vi "Load-Save Hardware Config.vi"(7 "Standalone ?":bool, 8 "error in":errorcluster, 9 "Hardware Configuration I/P":T1={"Dev. PC"=FALSE, "Swap XY on stage"=FALSE, "No of AOD"=0, "Computer MAC address"="", "Externalise Triggers"=FALSE, "Trigger HW config"={"Available Device List"=0, "Device Address"=""}, "DAQmx Chan"={"Pockels AO"="", "Hard shutter AO"="", "PMT AOs"="", "Galvo AOs"="", "Power meter AI"=""}, "XY stage available"=FALSE, "XY Stage"={"COM port"="", "Baudrate"=0, "Type"=""}, "Z stage available"=FALSE, "Z Stage config cluster"={"COM port"="COM7", "Baudrate"=0, "Type"=""}, "Encoder available"=FALSE, "Encoder"={"IP address"="224.0.1.103", "Port"=7000, "Wheel radius (cm)"=16.0, "Encoder Trigger"=""}, "VidRec available"=FALSE, "Cam VidRec"={"DO flag-Video record"="", "DO flag-Trial start"=""}, "Laser Power Control HW config"={"Laser Power Control"="", "Laser Power Modulation Control"=enum."NI"}, "Laser 1 available"=FALSE, "Laser 1 config cluster"={"COM port"="COM7", "Baud Rate"=0, "Type"=""}, "Prechirper 1 available"=FALSE, "Prechirper 1 config cluster"={"Type"="", "Baud Rate"=0, "COM port"="COM7"}, "Control system.FPGA available?"=FALSE, "Control Sys. HW config"={"Control system.FPGA Type"=enum."Virtex 5", "Control system.Network adapter name"="", "Control system.MAC address"="", "Control system.Ethernet Port"=0, "Control system.Ethernet Port Opened"=FALSE}, "DAQ FPGA HW Config"={"FGPA Ref"=refnum, "Target"="RIO0", "input card type"=enum."AC Card"}} {"Encoder"."Wheel radius (cm)" format="%#_13g"}, 11 "Function":T16=enum."Load from file") -> (0 "error out":errorcluster, 1 "Hardware Configuration O/P":T1={"Dev. PC"=FALSE, "Swap XY on stage"=FALSE, "No of AOD"=0, "Computer MAC address"="", "Externalise Triggers"=FALSE, "Trigger HW config"={"Available Device List"=0, "Device Address"=""}, "DAQmx Chan"={"Pockels AO"="", "Hard shutter AO"="", "PMT AOs"="", "Galvo AOs"="", "Power meter AI"=""}, "XY stage available"=FALSE, "XY Stage"={"COM port"="", "Baudrate"=0, "Type"=""}, "Z stage available"=FALSE, "Z Stage config cluster"={"COM port"="COM7", "Baudrate"=0, "Type"=""}, "Encoder available"=FALSE, "Encoder"={"IP address"="224.0.1.103", "Port"=7000, "Wheel radius (cm)"=16.0, "Encoder Trigger"=""}, "VidRec available"=FALSE, "Cam VidRec"={"DO flag-Video record"="", "DO flag-Trial start"=""}, "Laser Power Control HW config"={"Laser Power Control"="", "Laser Power Modulation Control"=enum."NI"}, "Laser 1 available"=FALSE, "Laser 1 config cluster"={"COM port"="COM7", "Baud Rate"=0, "Type"=""}, "Prechirper 1 available"=FALSE, "Prechirper 1 config cluster"={"Type"="", "Baud Rate"=0, "COM port"="COM7"}, "Control system.FPGA available?"=FALSE, "Control Sys. HW config"={"Control system.FPGA Type"=enum."Virtex 5", "Control system.Network adapter name"="", "Control system.MAC address"="", "Control system.Ethernet Port"=0, "Control system.Ethernet Port Opened"=FALSE}, "DAQ FPGA HW Config"={"FGPA Ref"=refnum, "Target"="RIO0", "input card type"=enum."AC Card"}} {"Encoder"."Wheel radius (cm)" format="%#_13g"})   [LabVIEW 2017]
uses:
  <vilib>/Utility/config.llb/NI_LVConfig.lvlib
  Typedefs/Which path.ctl
  Typedefs/XY Stage config cluster.ctl
  <vilib>/userdefined/High Color/nirio_resource_hc.ctl
  Typedefs/DAQmx physical channels cluster.ctl
  Typedefs/Save-Load enum.ctl
  Typedefs/FPGA input type AC-DC.ctl
  Typedefs/Encoder config cluster.ctl
  Typedefs/Cam VidRec HW config setup cluster.ctl
  Typedefs/Control Sys HW config cluster.ctl
  Typedefs/Z Stage config cluster.ctl
  Typedefs/Triggers HW config.ctl
  Typedefs/Laser 1 config cluster.ctl
  Typedefs/PreChirper 1 config cluster.ctl
  Typedefs/Laser Power Control HW config.ctl
  Typedefs/Hardware Configuration settings.ctl
  RIG-SPECIFIC FILES/FPGA Refs/FPGA Ref.ctl
  Typedefs/DAQ FPGA HW config cluster.ctl
panel:
  # "<--- The \"PMT AOs\" DAQmx string will always contain\n                       2 channels is this format: PXI1Slot4/ao2:3"
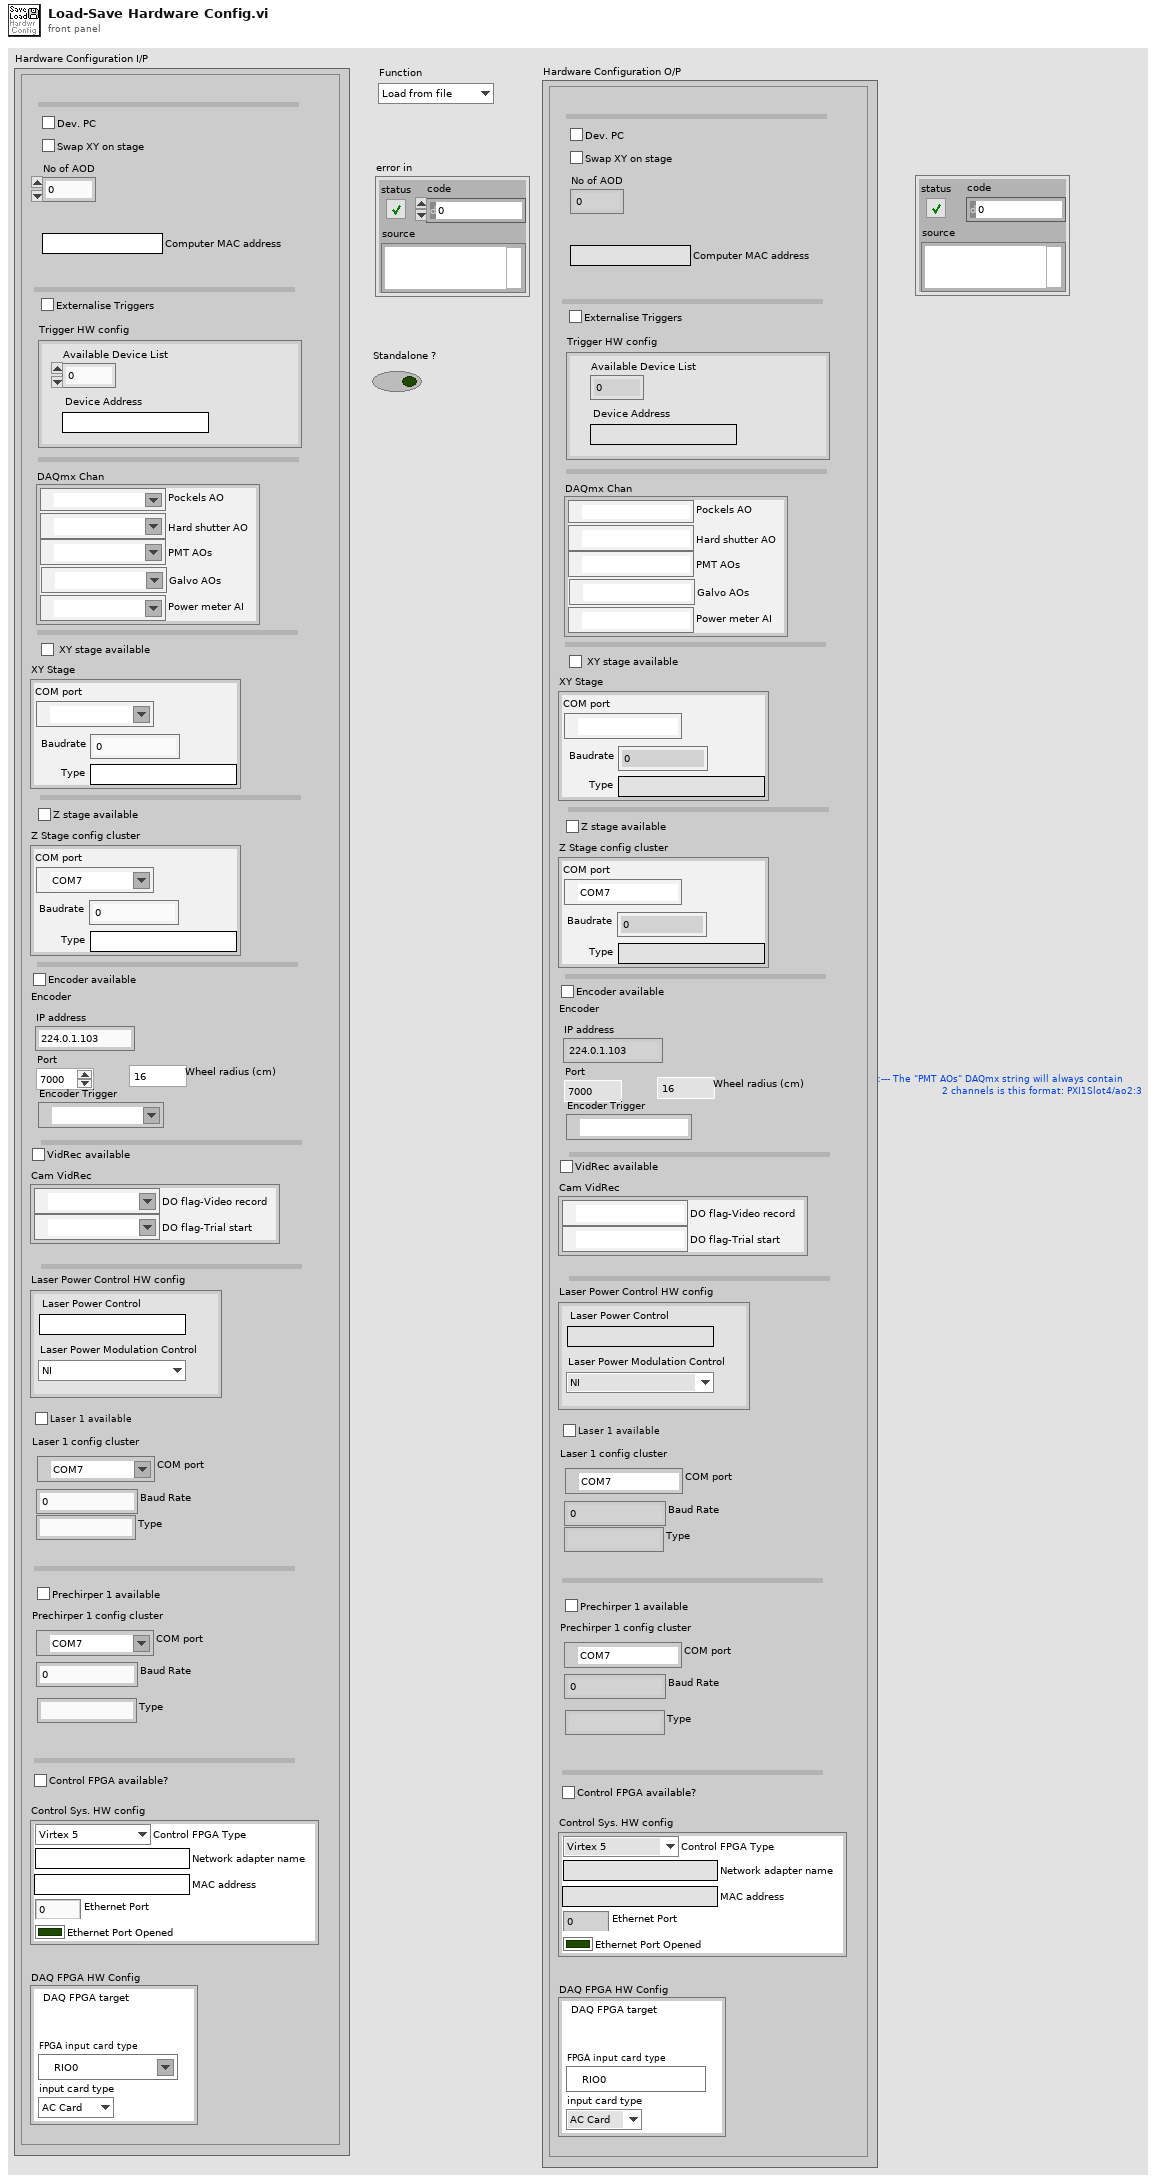
[diagram p1: front panel]
types:
  T1 = typedef "Hardware Configuration settings.ctl" = cluster{"Dev. PC":bool, "Swap XY on stage":bool, "No of AOD":u8, "Computer MAC address":string, "Externalise Triggers":bool, "Trigger HW config":T2, "DAQmx Chan":T3, "XY stage available":bool, "XY Stage":T4, "Z stage available":bool, "Z Stage config cluster":T5, "Encoder available":bool, "Encoder":T6, "VidRec available":bool, "Cam VidRec":T7, "Laser Power Control HW config":T8, "Laser 1 available":bool, "Laser 1 config cluster":T9, "Prechirper 1 available":bool, "Prechirper 1 config cluster":T10, "Control system.FPGA available?":bool, "Control Sys. HW config":T11, "DAQ FPGA HW Config":T12}
  T2 = typedef "Triggers HW config.ctl" = cluster{"Available Device List":i32, "Device Address":string}
  T3 = typedef "DAQmx physical channels cluster.ctl" = cluster{"Pockels AO":tag, "Hard shutter AO":tag, "PMT AOs":tag, "Galvo AOs":tag, "Power meter AI":tag}
  T4 = typedef "XY Stage config cluster.ctl" = cluster{"COM port":refnum<visa-resource-name>, "Baudrate":i32, "Type":string}
  T5 = typedef "Z Stage config cluster.ctl" = cluster{"COM port":refnum<visa-resource-name>, "Baudrate":i32, "Type":string}
  T6 = typedef "Encoder config cluster.ctl" = cluster{"IP address":string, "Port":u16, "Wheel radius (cm)":dbl, "Encoder Trigger":tag}
  T7 = typedef "Cam VidRec HW config setup cluster.ctl" = cluster{"DO flag-Video record":tag, "DO flag-Trial start":tag}
  T8 = typedef "Laser Power Control HW config.ctl" = cluster{"Laser Power Control":string, "Laser Power Modulation Control":enum16{"NI", "FPGA"}}
  T9 = typedef "Laser 1 config cluster.ctl" = cluster{"COM port":refnum<visa-resource-name>, "Baud Rate":i32, "Type":string}
  T10 = typedef "PreChirper 1 config cluster.ctl" = cluster{"Type":string, "Baud Rate":i32, "COM port":refnum<visa-resource-name>}
  T11 = typedef "Control Sys HW config cluster.ctl" = cluster{"Control system.FPGA Type":enum16{"Virtex 5", "Virtex 7"}, "Control system.Network adapter name":string, "Control system.MAC address":string, "Control system.Ethernet Port":u32, "Control system.Ethernet Port Opened":bool}
  T12 = typedef "DAQ FPGA HW config cluster.ctl" = cluster{"FGPA Ref":T13, "Target":T14, "input card type":T15}
  T13 = typedef "FPGA Ref.ctl" = refnum<k20>
  T14 = typedef "nirio_resource_hc.ctl" = tag
  T15 = typedef "FPGA input type AC-DC.ctl" = enum16{"AC Card", "DC Card"}
  T16 = typedef "Save-Load enum.ctl" = enum16{"Save to file", "Load from file", "Compare from file"}
  T17 = typedef "Which path.ctl" = enum16{"Configuration Files", "Calibration Files", "Images", "Setup.ini", "Loaded User profile.ini", "User's-Previous session.ini", "New user profile.ini", "Selected User profile.ini", "User profiles folder", "Power meter scaling.txt", "FOV Cal.ini", "Calibration.ini"}
  T18 = typedef "NI_LVConfig.lvlib/Config Data RefNum.ctl" = refnum<k1>
  T19 = typedef "Ini file interface (String).ctl" = cluster{"key":string, "Save?":bool, "Default":string}[]
  T20 = typedef "Ini file interface (DBL).ctl" = cluster{"key":string, "Save?":bool, "Default":dbl}[]
  T21 = typedef "Ini file interface (Boolean).ctl" = cluster{"key":string, "Save?":bool, "Default":bool}[]
  T22 = cluster{"key":string, "Save?":bool, "Default":dbl}
  T23 = cluster{"key":string, "Save?":bool, "Default":dbl}[]
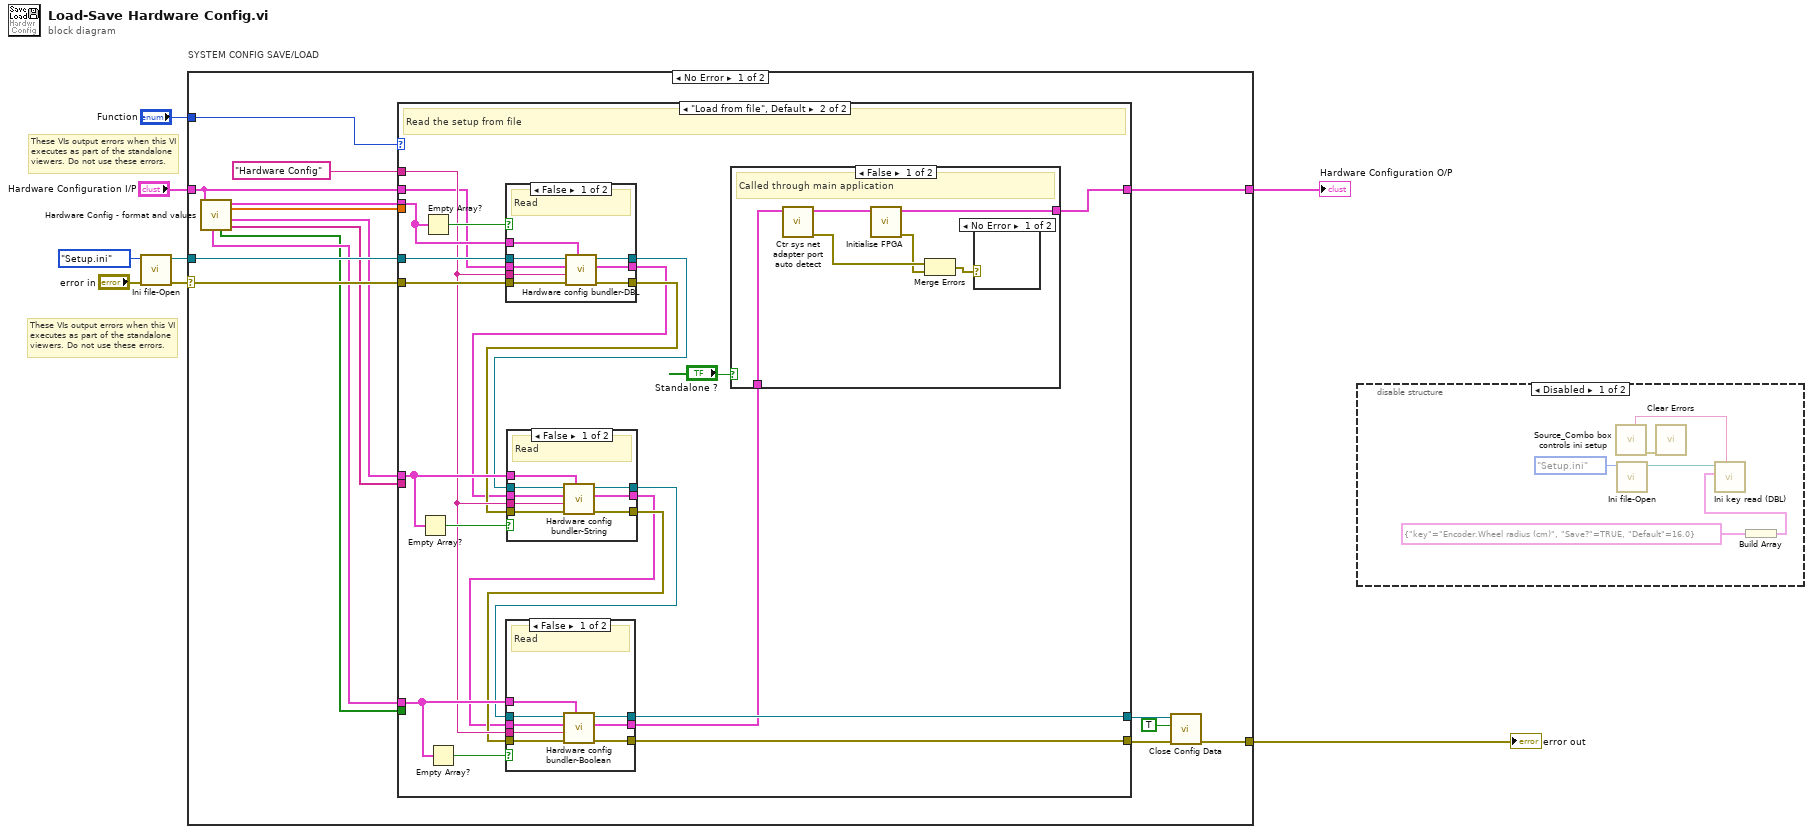
[diagram p0: block diagram]
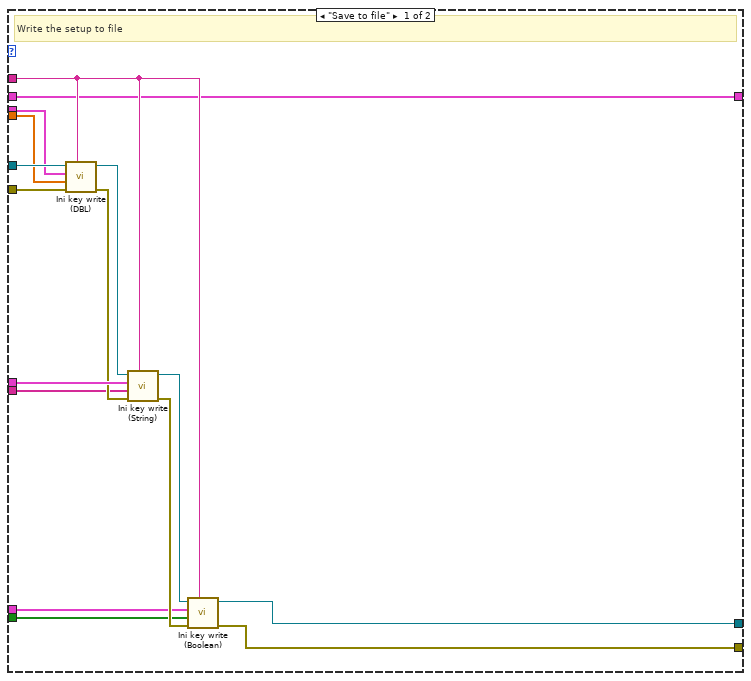
[diagram p3: hidden frame]
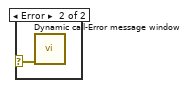
[diagram p4: hidden frame]
diagram:
  # "These VIs output errors when this VI executes as part of the standalone viewers. Do not use these errors."
  # "These VIs output errors when this VI executes as part of the standalone viewers. Do not use these errors."
  n1 = call "Ini file-Open.vi"("Error In"="error in", "Which file?"=Which_path."Setup.ini") -> ("error out"=w6:errorcluster, "User profile ini file ref"=w4:T18)  [unwired: 6 in, 2 out]
  n2 = case "SYSTEM CONFIG SAVE/LOAD" shown="No Error" w6 {
    selector: w6 -> [w20 w104]
    tunnel: [w18 w104] -> w3
    tunnel: "Hardware Configuration I/P" -> [w13 w103]
    tunnel: [w22 w103] -> w1
    tunnel: "Function" -> [w21 _]
    tunnel: w4 -> [w19 _]
    frame No Error {
      n3 = call "Hardware Config - format and values.vi"("Hardware Configuration"=w13) -> (0:"String"=w11:string[], 1:"String"=w12:T19, 2:"Numeric"=w14:dbl[], 3:"Numeric"=w15:T20, 4:"Boolean"=w9:bool[], 6:"Boolean"=w10:T21)  [unwired: 5 in]
      n4 = case shown="\"Load from file\", Default" w21 {
        tunnel: [w27 w56] -> w17
        tunnel: [w26 w57] -> w23
        tunnel: w20 -> [w39 w58]
        tunnel: w19 -> [w40 w61]
        tunnel: "Hardware Config" -> [w29 w51]
        tunnel: w15 -> [w37 w60]
        tunnel: w14 -> [w38 _]
        tunnel: w9 -> [w28 _]
        tunnel: w10 -> [w30 w55]
        tunnel: w11 -> [w33 _]
        tunnel: w12 -> [w36 w52]
        tunnel: [w25 w42] -> w22
        tunnel: w13 -> [w25 w46]
        frame "Save to file" {
          # "Write the setup to file"
          n5 = call "Ini key write (DBL).vi"("Section"=w29, "error in (no error)"=w39, "Values (DBL)"=w38, "Ini file interface"=w37, "Ini file refnum in"=w40) -> ("error out"=w34:errorcluster, "Ini file refnum out"=w35:T18)  [unwired: 5 in]
          n6 = call "Ini key write (String).vi"("Section"=w29, "error in (no error)"=w34, "Values (String)"=w33, "Ini file interface"=w36, "Ini file refnum in"=w35) -> ("error out"=w31:errorcluster, "Ini file refnum out"=w32:T18)  [unwired: 5 in]
          n7 = call "Ini key write (Boolean).vi"("Section"=w29, "error in (no error)"=w31, "Values (Boolean)"=w28, "Ini file interface"=w30, "Ini file refnum in"=w32) -> ("error out"=w27:errorcluster, "Ini file refnum out"=w26:T18)  [unwired: 5 in]
        }
        frame "Load from file", Default {
          # "Read the setup from file"
          n8 = Empty Array?(array=w52) -> (empty?=w53:bool)
          n9 = Empty Array?(array=w60) -> (empty?=w59:bool)
          n10 = Empty Array?(array=w55) -> (empty?=w54:bool)
          n11 = case shown="False" w59 {
            tunnel: w61 -> [w99 w102]
            tunnel: [w98 w102] -> w47
            tunnel: [w97 w101] -> w48
            tunnel: w58 -> [w96 w101]
            tunnel: w51 -> [w94 _]
            tunnel: w60 -> [w95 _]
            tunnel: w46 -> [w92 w100]
            tunnel: [w93 w100] -> w45
            frame False {
              # "Read"
              n12 = call "Hardware config bundler-DBL.vi"("Keys setup.DBL"=w95, "error in (no error)"=w96, "Section name"=w94, "Hardware Configuration"=w92, "Refnum in"=w99) -> ("error out"=w97:errorcluster, "output cluster"=w93:T1, "Refnum out"=w98:T18)  [unwired: 4 in]
            }
            frame True {
              # "No parametersof such type"
            }
          }
          n13 = case shown="False" w53 {
            tunnel: [w74 w80] -> w50
            tunnel: [w73 w79] -> w49
            tunnel: w52 -> [w76 _]
            tunnel: w47 -> [w77 w80]
            tunnel: w48 -> [w72 w79]
            tunnel: w51 -> [w75 _]
            tunnel: w45 -> [w71 w78]
            tunnel: [w70 w78] -> w44
            frame False {
              # "Read"
              n14 = call "Hardware config bundler-String.vi"("Keys setup.String"=w76, "error in (no error)"=w72, "Section name"=w75, "Hardware Configuration I/P"=w71, "Refnum in"=w77) -> ("error out"=w73:errorcluster, "Hardware Configuration O/P"=w70:T1, "Refnum out"=w74:T18)  [unwired: 4 in]
            }
            frame True {
              # "No parametersof such type"
            }
          }
          n15 = case shown="False" w54 {
            tunnel: [w87 w91] -> w57
            tunnel: [w86 w90] -> w56
            tunnel: w55 -> [w83 _]
            tunnel: w50 -> [w88 w91]
            tunnel: w49 -> [w85 w90]
            tunnel: w51 -> [w84 _]
            tunnel: w44 -> [w81 w89]
            tunnel: [w82 w89] -> w43
            frame False {
              # "Read"
              n16 = call "Hardware config bundler-Boolean.vi"("Keys setup.Boolean"=w83, "error in (no error)"=w85, "Section name"=w84, "Hardware Configuration I/P"=w81, "Refnum in"=w88) -> ("error out"=w86:errorcluster, "Hardware Configuration O/P"=w82:T1, "Refnum out"=w87:T18)  [unwired: 4 in]
            }
            frame True {
              # "No parametersof such type"
            }
          }
          n17 = case shown="False" "Standalone ?" {
            tunnel: [w63 w69] -> w42
            tunnel: w43 -> [w62 w69]
            frame False {
              # "Called through main application"
              n18 = call "Ctr sys net adapter port auto detect.vi"("HW Config IN"=w62) -> ("error out"=w66:errorcluster, "HW config OUT"=w67:T1)  [unwired: 9 in]
              n19 = call "Initialise FPGA.vi"("Hardware Resources in"=w67) -> ("error out"=w65:errorcluster, "Hardware Resources out"=w63:T1)  [unwired: 9 in]
              n20 = Merge Errors(w66, w65) -> (w64:errorcluster)
              n21 = case shown="No Error" w64 {
                selector: w64 -> [_ w68]
                frame No Error {
                }
                frame Error {
                  n22 = call "Dynamic call-Error message window.vi"("error in (no error)"=w68) -> ()  [unwired: 10 in, 1 out]
                }
              }
            }
            frame True {
              # "Standalone viewer"
            }
          }
        }
      }
      n23 = call <vilib>:"Close Config Data.vi"("error in (no error)"=w17, "write file if changed (T)"=TRUE ("write configuration file? (F)"), "refnum"=w23) -> ("error out"=w18:errorcluster)  [unwired: 7 in, 1 out]
    }
    frame Error {
    }
  }
  "error out" <- w3
  "Hardware Configuration O/P" <- w1
  n24 = disable-structure shown="Disabled" {
    frame Disabled {
      n25 = call "Source_Combo box controls ini setup.vi"() -> ("error out"=w105:errorcluster, "Section name"=w106:string)  [unwired: 9 in, 1 out]
      n26 = call "Ini file-Open.vi"("Which file?"=Which_path."Setup.ini") -> ("User profile ini file ref"=w109:T18)  [unwired: 7 in, 3 out]
      n27 = call <vilib>:"Clear Errors.vi"("error in (no error)"=w105) -> ()  [unwired: 5 in, 2 out]
      n28 = Build Array(T22 {"key"="Encoder.Wheel radius (cm)", "Save?"=TRUE, "Default"=16.0}) -> (w107:T23)
      n29 = call "Ini key read (DBL).vi"("Section name"=w106, "Parameter names & setup"=w107, "Ini file refnum in"=w109) -> ()  [unwired: 6 in, 3 out]
    }
    frame Enabled {
    }
  }
